vi "Get SW Version.vi"(8 "error in (no error)":errorcluster, 11 "Current VI's Path":path) -> (0 "error out":errorcluster, 3 "FileVersion":string)   [LabVIEW 2015]
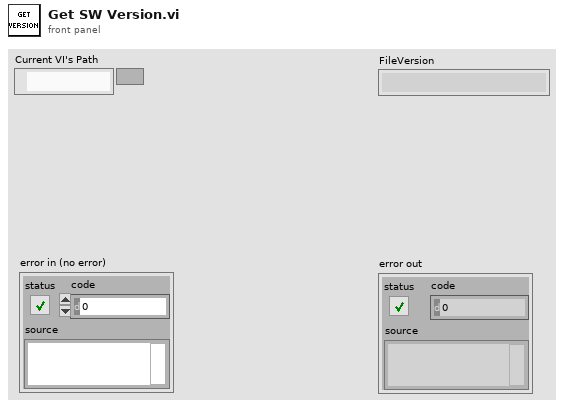
[diagram p1: front panel]
types:
  T1 = enum32{"invalid app kind", "Development System", "Run Time System", "Student Edition", "Embedded LabVIEW", "Evaluation", "Custom"}
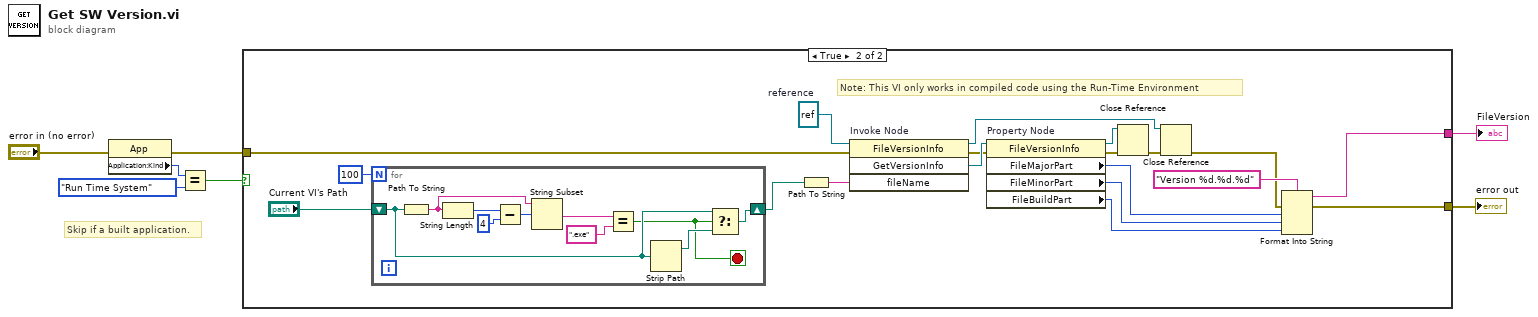
[diagram p0: block diagram]
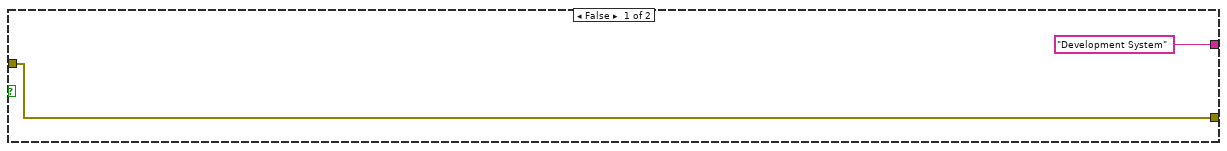
[diagram p2: hidden frame]
diagram:
  # "Skip if a built application."
  n1 = property class="App"(error in="error in (no error)") -> (error out=w1:errorcluster, "Application:Kind"=w6:T1)  [unwired: 1 in, 1 out]
  n2 = Equal?(x=w6, y=T1."Run Time System" ("Application:Kind")) -> (x = y?=w3:bool)
  n3 = case shown="True" w3 {
    tunnel: w1 -> [w9 w15]
    tunnel: [w9 w14] -> w7
    tunnel: ["Development System" ("format string") w13] -> w4
    frame False {
    }
    frame True {
      w28 = refnum<k24> refnum  # reference
      # "Note: This VI only works in compiled code using the Run-Time Environment"
      n4 = for {
        N: 100 -> [_]
        shift-right: [w31] -> w12
        shift-left: "Current VI's Path" -> [w30]
        stop <- w29 stop-if-true
        n5 = Path To String(path=w30) -> (string=w35:string)
        n6 = String Length(string=w35) -> (length=w38:i32)
        n7 = Subtract(x=w38, y=4) -> (x-y=w37:i32)
        n8 = String Subset(string=w35, offset (0)=w37) -> (substring=w34:string)  [unwired: 1 in]
        n9 = Equal?(x=w34, y=".exe") -> (x = y?=w29:bool)
        n10 = Strip Path(path=w30) -> (stripped path=w32:path)  [unwired: 1 out]
        n11 = Select(t=w30, s=w29, f=w32) -> (s? t:f=w31:path)
      }
      n12 = Path To String(path=w12) -> (string=w27:string)
      n13 = invoke on="Invoke Node" class="FileVersionInfo" method="GetVersionInfo"(reference=w28, error in=w15, "fileName"=w27) -> (reference out=w21:refnum<k24>, error out=w25:errorcluster, "GetVersionInfo"=w26:refnum<k24>)  [unwired: 1 in, 1 out]
      n14 = property on="Property Node" class="FileVersionInfo"(reference=w26, error in=w25) -> (reference out=w24:refnum<k24>, error out=w23:errorcluster, "FileMajorPart"=w17:i32, "FileMinorPart"=w19:i32, "FileBuildPart"=w18:i32)
      n15 = Close Reference(reference=w24, error in (no error)=w23) -> (error out=w22:errorcluster)
      n16 = Close Reference(reference=w21, error in (no error)=w22) -> (error out=w16:errorcluster)
      n17 = Format Into String(format string="Version %d.%d.%d", error in=w16, w17, w19, w18) -> (resulting string=w13:string, error out=w14:errorcluster)  [unwired: 1 in]
    }
  }
  "error out" <- w7
  "FileVersion" <- w4
